vi "烧录座设定界面.vi"(8 "错误输入（无错误）":errorcluster, 10 "界面切换队列":refnum<queue>, 11 "VISA资源名称输入":refnum<visa-resource-name>) -> (0 "错误输出":errorcluster, 3 "VISA资源名称输出":refnum<visa-resource-name>)   [LabVIEW 2018]
panel:
  out "毫秒计时值":u32
  in  "枚举":T1(ring)
  in  "选项卡控件":enum32{"选项卡 1", "选项卡 2"}(tab)
  out "烧录座显示界面":bool
  out "读DDT32670+写R57F":dbl
  out "读DDT32668+写R57E":dbl
  out "读DDT32666+写R57D":dbl
  out "读DDT32664+写R57C":dbl
  out "读DDT32662+写R57B":dbl
  out "读DDT32660+写R57A":dbl
  out "读DDT32658+写R579":dbl
  out "读DDT32656+写R578":dbl
  out "读DDT32654+写R577":dbl
  out "读DDT32652+写R576":dbl
  out "读DDT32650+写R575":dbl
  out "读DDT32648+写R574":dbl
  out "读DDT32646+写R573":dbl
  out "读DDT32644+写R572":dbl
  out "读DDT32642+写R571":dbl
  out "读DDT32640+写R570":dbl
  out "写DDT32569":dbl
  out "写DDT32594":dbl
  out "DDT90356":dbl
  out "DDT90348":dbl
  out "自动界面":bool
  out "手动界面":bool
  out "参数界面":bool
  out "IO界面":bool
  out "产品界面":bool
  out "字符串":string
  out "DDT90352":dbl
  out "DDT90360":dbl
  out "通讯周期":dbl
  out "DT1184":T2(ring)
  # "X"
  # "Z1"
  # "Z2"
  # "Y"
  # "烧录座使用寿命"
  # "次"
  # "次"
  # "烧录座连续NG次数"
  # "烧录座当前烧录次数"
  # "1"
  # "2"
  # "3"
  # "4"
  # "5"
  # "6"
  # "7"
  # "8"
  # "9"
  # "10"
  # "12"
  # "14"
  # "15"
  # "16"
  # "11"
  # "13"
  # "鼠标点击数值框清零"
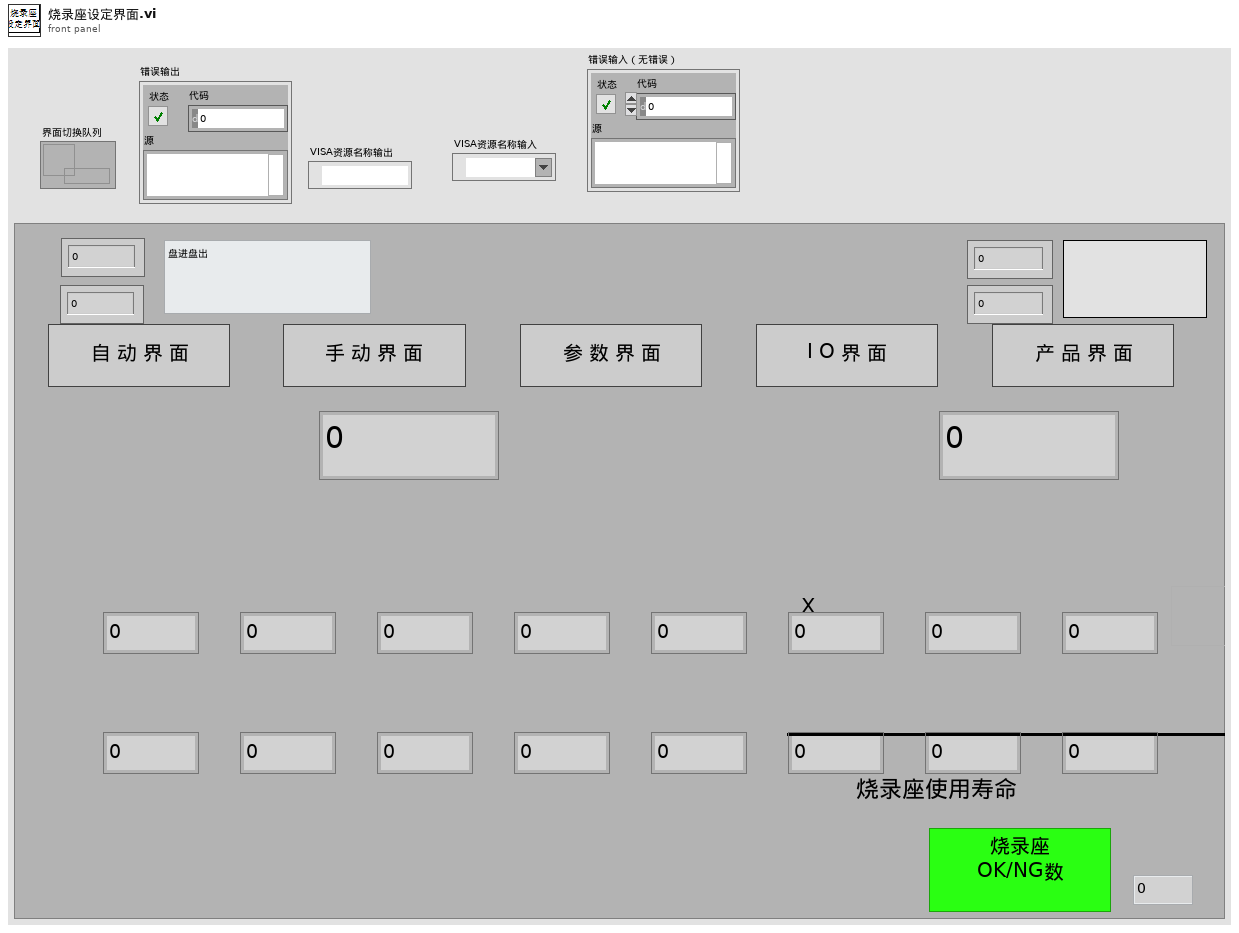
[diagram p1: front panel]
types:
  T1 = enum16{"读初始化", "读DDT32640+5", "读DDT32650+5", "读DDT32660+5", "读DDT32670", "读DDT32594", "读DDT32569", "读DDT90356", "读DT1184", "读DDT90348", ""}
  T2 = enum16{"盘进盘出", "卷进卷出", "盘进卷出", "管进盘出", "管进卷出", "卷进盘出", ""}
  T3 = enum8{"Enabled", "Disabled", "Disabled and Grayed Out"}
  T4 = typedef "数据簇.ctl" = cluster{"字符串":string, "数值":i32, "布尔":bool}
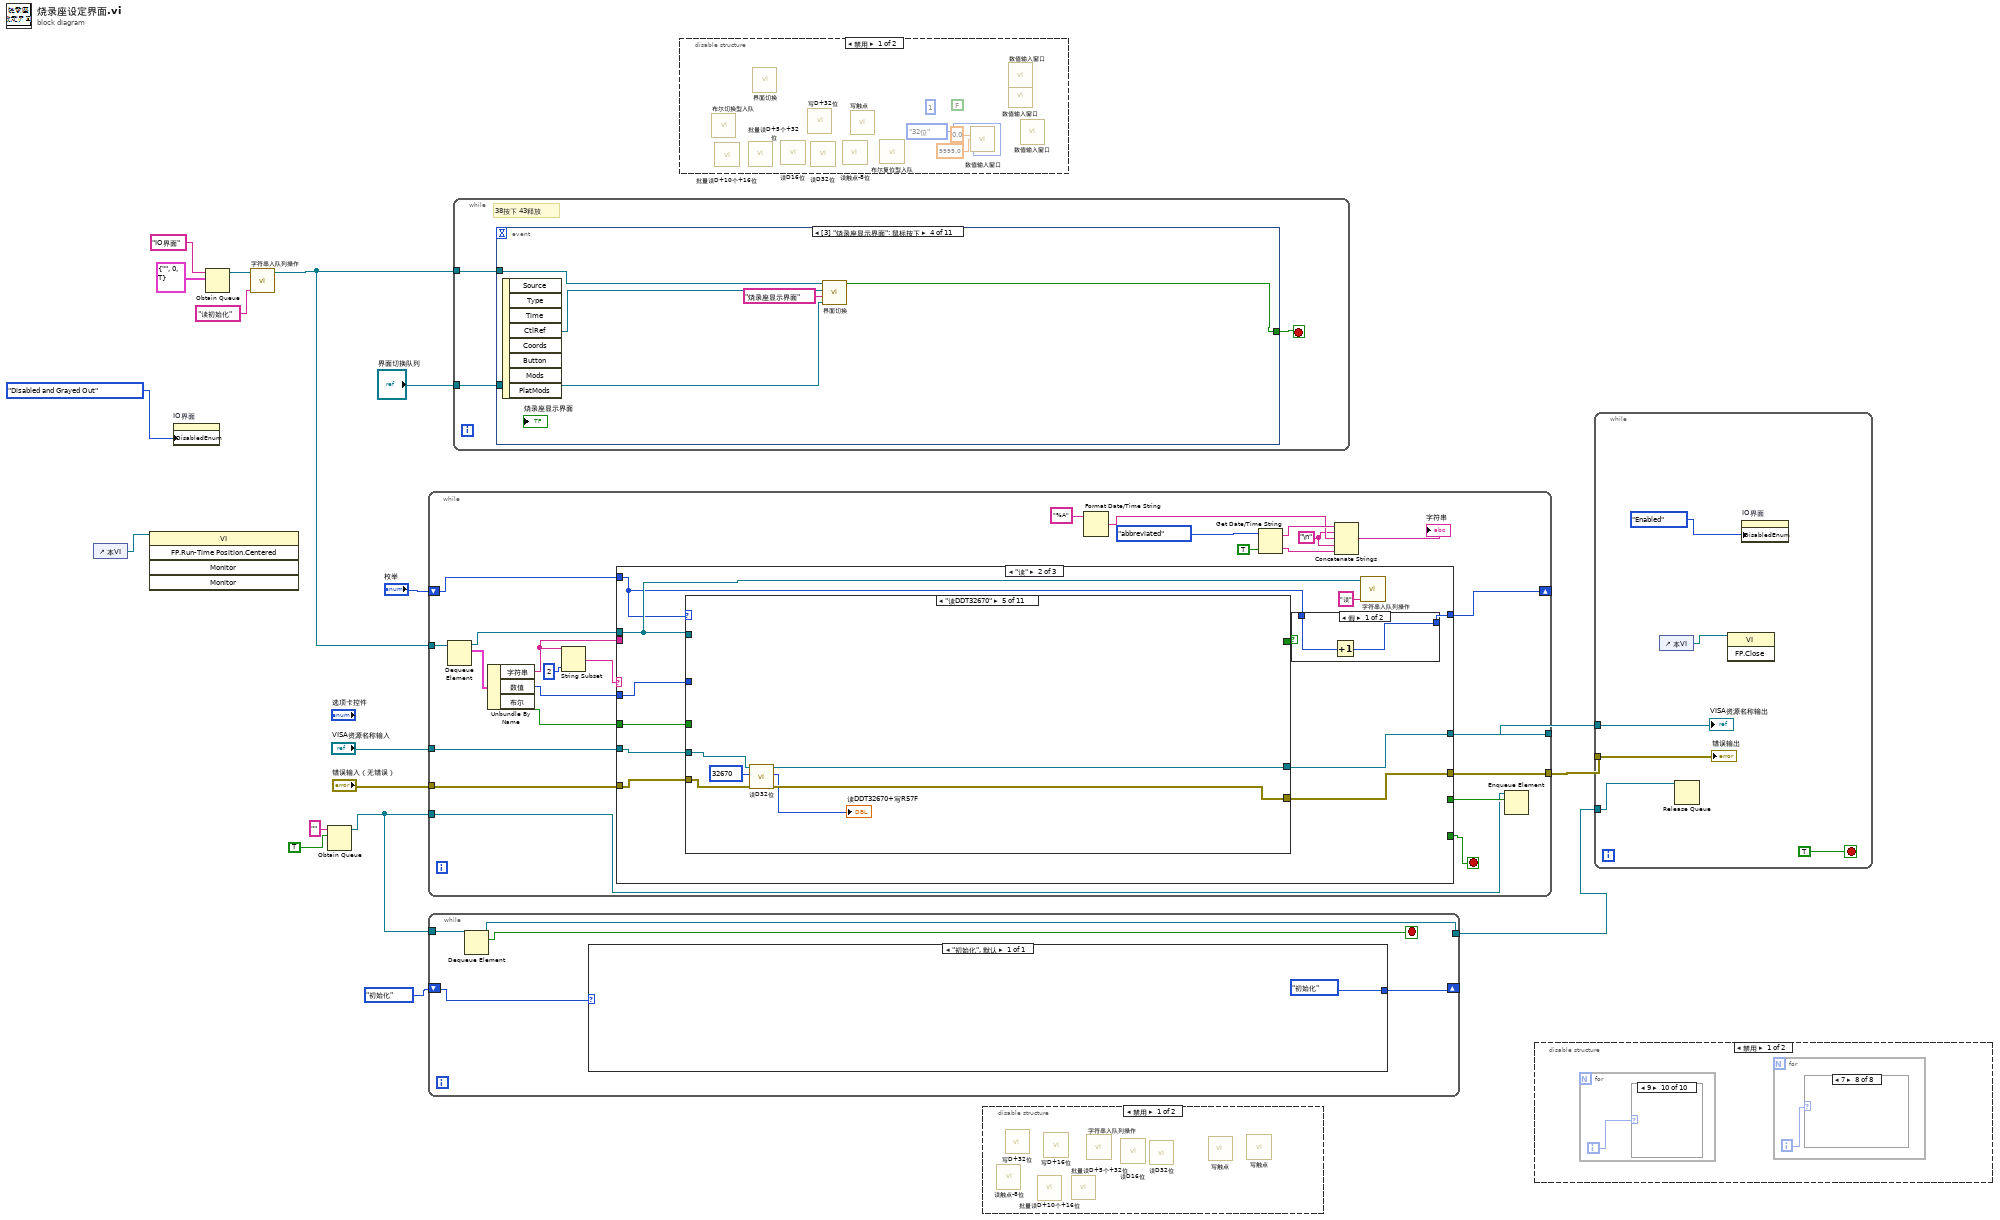
[diagram p0: block diagram]
diagram:
  n1 = control-ref of="本VI"() -> (w1:refnum<vi>)
  n2 = invoke class="VI" method="FP.Run-Time Position.Centered"(reference=w1) -> ()  [unwired: 4 in, 5 out]
  n3 = property on="IO界面" class="Bool"("DisabledEnum"=T3."Disabled and Grayed Out" ("禁用")) -> ()  [unwired: 2 in, 2 out]
  n4 = Obtain Queue(name (unnamed)="IO界面" ("名称（未命名）"), element data type=T4 {"字符串"="", "数值"=0, "布尔"=TRUE}) -> (queue out=w11:refnum<queue>)  [unwired: 3 in, 2 out]
  n5 = call "字符串入队列操作.vi"("字符消息入队列"="读初始化", "界面切换队列"=w11) -> ("队列输出"=w3:refnum<queue>)  [unwired: 9 in]
  n6 = Obtain Queue(name (unnamed)="" ("名称（未命名）"), element data type=TRUE) -> (queue out=w6:refnum<queue>)  [unwired: 3 in, 2 out]
  n7 = while {
    tunnel: w3 -> [w39]
    tunnel: "VISA资源名称输入" -> [w32]
    tunnel: "错误输入（无错误）" -> [w31]
    tunnel: [w30] -> w13
    tunnel: [w29] -> w12
    shift-right: [w26] -> _
    shift-left: "枚举" -> [w27]
    tunnel: w6 -> [w19]
    stop <- w21 stop-if-true
    w23 = "\n"
    n8 = Dequeue Element(queue=w39) -> (queue out=w36:refnum<queue>, element=w38:T4)  [unwired: 2 in, 2 out]
    n9 = Unbundle By Name(w38) -> ("字符串"=w33:string, "数值"=w35:i32, "布尔"=w34:bool)
    n10 = String Subset(string=w33, length (rest)=2 ("长度（剩余）")) -> (substring=w37:string)  [unwired: 1 in]
    n11 = case shown="\"读\"" w37 {
      selector: w37 -> [w46 _ _]
      tunnel: w36 -> [_ w54 w180]
      tunnel: w35 -> [_ w61 w179]
      tunnel: w34 -> [_ w60 w178]
      tunnel: w33 -> [_ _ w172]
      tunnel: w32 -> [w45 w59 w177]
      tunnel: w31 -> [w44 w58 w176]
      tunnel: [w45 w57 w174] -> w30
      tunnel: [w44 w56 w173] -> w29
      tunnel: [_ _ w175] -> w21
      tunnel: w27 -> [_ w52 _]
      tunnel: [_ w51 _] -> w26
      tunnel: [_ _ w170] -> w20
      frame "", Default {
        n12 = Concatenate Strings("无对应消息分支**" ("消息"), w46, "**" ("字符串"), "读写状态机" ("字符串")) -> (w48:string)
        n13 = One Button Dialog(message=w48) -> ()  [unwired: 1 in, 1 out]
      }
      frame "读" {
        n14 = case shown="\"读DDT32670\"" w52 {
          tunnel: w54 -> [_ _ _ _ _ _ _ _ _ _ _]
          tunnel: w61 -> [_ _ _ _ _ _ _ _ _ _ _]
          tunnel: w59 -> [w66 w72 w85 w98 w111 w117 w123 w135 w144 w157 w169]
          tunnel: w58 -> [w65 w71 w84 w97 w110 w116 w122 w134 w143 w156 w168]
          tunnel: [w66 w70 w83 w95 w109 w115 w120 w133 w142 w155 w169] -> w57
          tunnel: [w65 w69 w82 w94 w108 w114 w119 w132 w141 w154 w168] -> w56
          tunnel: w60 -> [_ _ _ _ _ _ _ _ _ _ _]
          tunnel: [_ _ _ _ _ _ _ _ _ _ TRUE] -> w53
          frame "读初始化" {
            n15 = Tick Count (ms)() -> (millisecond timer value=→"毫秒计时值":u32)
          }
          frame "读DDT32640+5" {
            n16 = call "批量读D+5个+32位.vi"("error out"=w71, "读取D地址"=32640, "VISA resource name out"=w72) -> ("error IO"=w69:errorcluster, "数组"=w67:i32[], "VISA resource name out 2"=w70:refnum<visa-resource-name>)  [unwired: 5 in, 1 out]
            n17 = for {
              tunnel: w67 -> [w73] mode=indexing
              i -> [w74]
              n18 = case shown="4" w74 {
                tunnel: w73 -> [w75 w76 w77 w78 w79]
                frame 0, Default {
                  "读DDT32640+写R570" <- w75
                }
                frame 1 {
                  "读DDT32642+写R571" <- w76
                }
                frame 2 {
                  "读DDT32644+写R572" <- w77
                }
                frame 3 {
                  "读DDT32646+写R573" <- w78
                }
                frame 4 {
                  "读DDT32648+写R574" <- w79
                }
              }
            }
          }
          frame "读DDT32650+5" {
            n19 = call "批量读D+5个+32位.vi"("error out"=w84, "读取D地址"=32650, "VISA resource name out"=w85) -> ("error IO"=w82:errorcluster, "数组"=w80:i32[], "VISA resource name out 2"=w83:refnum<visa-resource-name>)  [unwired: 5 in, 1 out]
            n20 = for {
              tunnel: w80 -> [w86] mode=indexing
              i -> [w87]
              n21 = case shown="3" w87 {
                tunnel: w86 -> [w88 w89 w90 w91 w92]
                frame 0, Default {
                  "读DDT32650+写R575" <- w88
                }
                frame 1 {
                  "读DDT32652+写R576" <- w89
                }
                frame 2 {
                  "读DDT32654+写R577" <- w90
                }
                frame 3 {
                  "读DDT32656+写R578" <- w91
                }
                frame 4 {
                  "读DDT32658+写R579" <- w92
                }
              }
            }
          }
          frame "读DDT32660+5" {
            n22 = call "批量读D+5个+32位.vi"("error out"=w97, "读取D地址"=32660, "VISA resource name out"=w98) -> ("error IO"=w94:errorcluster, "数组"=w93:i32[], "VISA resource name out 2"=w95:refnum<visa-resource-name>)  [unwired: 5 in, 1 out]
            n23 = for {
              tunnel: w93 -> [w99] mode=indexing
              i -> [w100]
              n24 = case shown="0, 默认" w100 {
                tunnel: w99 -> [w101 w102 w103 w104 w105]
                frame 0, Default {
                  "读DDT32660+写R57A" <- w101
                }
                frame 1 {
                  "读DDT32662+写R57B" <- w102
                }
                frame 2 {
                  "读DDT32664+写R57C" <- w103
                }
                frame 3 {
                  "读DDT32666+写R57D" <- w104
                }
                frame 4 {
                  "读DDT32668+写R57E" <- w105
                }
              }
            }
          }
          frame "读DDT32670" {
            n25 = call "读D32位.vi"("error out"=w110, "读取D地址"=32670, "VISA resource name out"=w111) -> ("error IO"=w108:errorcluster, "数值"=→"读DDT32670+写R57F":i32, "VISA resource name out 2"=w109:refnum<visa-resource-name>)  [unwired: 6 in]
          }
          frame "读DDT32594" {
            n26 = call "读D32位.vi"("error out"=w116, "读取D地址"=32594, "VISA resource name out"=w117) -> ("error IO"=w114:errorcluster, "数值"=→"写DDT32594":i32, "VISA resource name out 2"=w115:refnum<visa-resource-name>)  [unwired: 6 in]
          }
          frame "读DDT32569" {
            n27 = call "读D32位.vi"("error out"=w122, "读取D地址"=32569, "VISA resource name out"=w123) -> ("error IO"=w119:errorcluster, "数值"=→"写DDT32569":i32, "VISA resource name out 2"=w120:refnum<visa-resource-name>)  [unwired: 6 in]
          }
          frame "读DDT90356" {
            n28 = call "批量读D+5个+32位.vi"("error out"=w134, "读取D地址"=90356, "VISA resource name out"=w135) -> ("error IO"=w132:errorcluster, "数组"=w138:i32[], "VISA resource name out 2"=w133:refnum<visa-resource-name>)  [unwired: 5 in, 1 out]
            n29 = Index Array(array=w138, index #1=0 ("索引"), index #2=2 ("索引")) -> (element #1=w131:i32, element #2=w130:i32)
            n30 = To Double Precision Float(number=w131) -> (double precision float=w129:dbl)
            n31 = To Double Precision Float(number=w130) -> (double precision float=w126:dbl)
            n32 = Divide(x=w129, y=100.0) -> (x/y=→"DDT90356":dbl)
            n33 = Divide(x=w126, y=100.0) -> (x/y=→"DDT90360":dbl)
          }
          frame "读DT1184" {
            n34 = call "读D16位.vi"("error out"=w143, "读取D地址"=1184, "VISA resource name out"=w144) -> ("error IO"=w141:errorcluster, "数值"=→"DT1184":u32, "VISA resource name out 2"=w142:refnum<visa-resource-name>)  [unwired: 5 in, 1 out]
          }
          frame "读DDT90348" {
            n35 = call "批量读D+5个+32位.vi"("error out"=w156, "读取D地址"=90348, "VISA resource name out"=w157) -> ("error IO"=w154:errorcluster, "数组"=w161:i32[], "VISA resource name out 2"=w155:refnum<visa-resource-name>)  [unwired: 5 in, 1 out]
            n36 = Index Array(array=w161, index #1=0 ("索引"), index #2=2 ("索引")) -> (element #1=w153:i32, element #2=w152:i32)
            n37 = To Double Precision Float(number=w152) -> (double precision float=w147:dbl)
            n38 = To Double Precision Float(number=w153) -> (double precision float=w151:dbl)
            n39 = Divide(x=w147, y=100.0) -> (x/y=→"DDT90352":dbl)
            n40 = Divide(x=w151, y=100.0) -> (x/y=→"DDT90348":dbl)
          }
          frame "" {
            n41 = local read "毫秒计时值"() -> (w165:u32)
            n42 = Tick Count (ms)() -> (millisecond timer value=w166:u32)
            n43 = Subtract(x=w166, y=w165) -> (x-y=w164:u32)
            n44 = Divide(x=w164, y=u32 1000) -> (x/y=→"通讯周期":dbl)
          }
        }
        n45 = case shown="假" w53 {
          tunnel: w52 -> [w63 _]
          tunnel: [w62 _] -> w51
          frame False {
            n46 = Increment(x=w63) -> (x+1=w62:T1)
          }
          frame True {
          }
        }
        n47 = call "字符串入队列操作.vi"("字符消息入队列"="读", "界面切换队列"=w54) -> ()  [unwired: 9 in, 1 out]
      }
      frame "写" {
        n48 = call "状态匹配.vi"("输入状态"=w172) -> ("输出状态"=w171:string)  [unwired: 10 in]
        n49 = case shown="\"写退出\"" w171 {
          selector: w171 -> [w183 _ _ _ _]
          tunnel: w180 -> [_ _ _ _ w223]
          tunnel: w179 -> [_ w189 w206 _ _]
          tunnel: w178 -> [_ _ _ w217 _]
          tunnel: w177 -> [w182 w199 w210 w222 w228]
          tunnel: w176 -> [w181 w198 w209 w221 w227]
          tunnel: [_ _ _ _ w226] -> w175
          tunnel: [w182 w197 w208 w220 w228] -> w174
          tunnel: [w181 w196 w207 w219 w227] -> w173
          tunnel: w172 -> [_ w188 w200 w211 _]
          tunnel: [_ _ _ _ w226] -> w170
          frame "", Default {
            n50 = Concatenate Strings("无对应消息分支**" ("消息"), w183, "**" ("字符串"), "写状态机" ("字符串")) -> (w187:string)
            n51 = One Button Dialog(message=w187) -> ()  [unwired: 1 in, 1 out]
          }
          frame "写DT" {
            n52 = String Length(string=w188) -> (length=w194:i32)
            n53 = Subtract(x=w194, y=4) -> (x-y=w192:i32)
            n54 = String Subset(string=w188, offset (0)=4 ("偏移量(0)"), length (rest)=w192) -> (substring=w191:string)
            n55 = Decimal String To Number(string=w191) -> (number=w190:i32)  [unwired: 2 in, 1 out]
            n56 = call "写D+16位.vi"("error out"=w198, "输入数值"=w189, "输入地址D"=w190, "VISA resource name out"=w199) -> ("error out 2"=w196:errorcluster, "VISA resource name out 2"=w197:refnum<visa-resource-name>)  [unwired: 3 in, 3 out]
          }
          frame "写DDT" {
            n57 = String Length(string=w200) -> (length=w204:i32)
            n58 = Subtract(x=w204, y=5) -> ()  [unwired: 1 out]
            n59 = String Subset(string=w200, offset (0)=5 ("偏移量(0)")) -> (substring=w201:string)  [unwired: 1 in]
            n60 = Decimal String To Number(string=w201) -> (number=w202:i32)  [unwired: 2 in, 1 out]
            n61 = call "写D+32位.vi"("error out"=w209, "输入数值"=w206, "输入地址D"=w202, "VISA resource name out"=w210) -> ("error out 2"=w207:errorcluster, "VISA resource name out 2"=w208:refnum<visa-resource-name>)  [unwired: 4 in, 2 out]
          }
          frame "写R" {
            n62 = String Length(string=w211) -> (length=w215:i32)
            n63 = Subtract(x=w215, y=3) -> (x-y=w213:i32)
            n64 = String Subset(string=w211, offset (0)=3 ("偏移量(0)"), length (rest)=w213) -> (substring=w212:string)
            n65 = call "写触点.vi"("布尔"=w217, "error out"=w221, "触点类型"="R", "写入起始地址"=w212, "VISA resource name out"=w222) -> ("error IO"=w219:errorcluster, "VISA resource name out 2"=w220:refnum<visa-resource-name>)  [unwired: 4 in, 1 out]
          }
          frame "写退出" {
            w226 = TRUE
            n66 = Flush Queue(queue=w223) -> (queue out=w224:refnum<queue>, error out=w225:errorcluster)  [unwired: 1 in, 1 out]
            n67 = Release Queue(queue=w224, error in (no error)=w225) -> ()  [unwired: 1 in, 3 out]
          }
        }
      }
    }
    n68 = Format Date/Time String(time format string (%c)="%A" ("时间格式字符串(%c)")) -> (date/time string=w24:string)  [unwired: 2 in]
    n69 = Get Date/Time String(date format (0)=enum16{"short", "long", "abbreviated"}."abbreviated" ("日期格式(0)"), want seconds? (F)=TRUE ("需要秒？(F)")) -> (date string=w41:string, time string=w22:string)  [unwired: 1 in]
    n70 = Concatenate Strings(w41, w23, w24, w23, w22) -> (→"字符串":string)
    n71 = Enqueue Element(queue=w19, element=w20) -> ()  [unwired: 2 in, 3 out]
  }
  n72 = while {
    shift-right: [w232] -> _
    shift-left: enum16{"初始化"}."初始化" -> [w233]
    tunnel: w6 -> [w231]
    tunnel: [w229] -> w5
    stop <- w230 stop-if-true
    n73 = Dequeue Element(queue=w231) -> (queue out=w229:refnum<queue>, element=w230:bool)  [unwired: 2 in, 2 out]
    n74 = case shown="\"初始化\", 默认" w233 {
      tunnel: [enum16{"初始化"}."初始化"] -> w232
      frame "初始化", Default {
      }
    }
  }
  n75 = while {
    tunnel: w3 -> [w236]
    tunnel: "界面切换队列" -> [w235]
    stop <- w237 stop-if-true
    # "38按下 43释放"
    n76 = event shown="[3] \"烧录座显示界面\": 鼠标按下" {
      selector: _ -> [_ _ _ _ _ _ _ _ _ _ _]
      dyn-events: _ -> [_ _ _ _ _ _ _ _ _ _ _]
      timeout: _ -> [_ _ _ _ _ _ _ _ _ _ _]
      tunnel: [w241 w243 w248 w253 _ _ _ w296 w301 _ w308] -> w237
      tunnel: w236 -> [w242 w247 w252 w257 w265 w273 w277 w300 w305 _ w307]
      tunnel: w235 -> [w240 w246 w251 w255 _ _ _ w299 w304 _ w306]
      event "IO界面": Mouse Down {
        n77 = event-data() -> ("CtlRef"=w239:refnum<vi>)  [unwired: 1 in, 7 out]
        n78 = call "界面切换.vi"("界面切换队列输入"=w240, "切换界面名称输入"="IO界面", "Bool引用句柄"=w239, "状态转移输入"=w242) -> ("布尔"=w241:bool)  [unwired: 7 in]
      }
      event "参数界面": Mouse Down {
        n79 = event-data() -> ("CtlRef"=w245:refnum<vi>)  [unwired: 1 in, 7 out]
        n80 = call "界面切换.vi"("界面切换队列输入"=w246, "切换界面名称输入"="参数界面", "Bool引用句柄"=w245, "状态转移输入"=w247) -> ("布尔"=w243:bool)  [unwired: 7 in]
      }
      event "产品界面": Mouse Down {
        n81 = event-data() -> ("CtlRef"=w250:refnum<vi>)  [unwired: 1 in, 7 out]
        n82 = call "界面切换.vi"("界面切换队列输入"=w251, "切换界面名称输入"="产品界面", "Bool引用句柄"=w250, "状态转移输入"=w252) -> ("布尔"=w248:bool)  [unwired: 7 in]
      }
      event "烧录座显示界面": Mouse Down {
        n83 = event-data() -> ("CtlRef"=w256:refnum<vi>)  [unwired: 1 in, 7 out]
        n84 = call "界面切换.vi"("界面切换队列输入"=w255, "切换界面名称输入"="烧录座显示界面", "Bool引用句柄"=w256, "状态转移输入"=w257) -> ("布尔"=w253:bool)  [unwired: 7 in]
      }
      event "写DDT32594": Mouse Down {
        n85 = event-data() -> ("CtlRef"=w262:refnum<vi>)  [unwired: 1 in, 7 out]
        n86 = call "数值输入窗口.vi"("消息入队"=w265, "字符串"="烧录座使用寿命次数", "字符消息入队列"="写DDT32594", "输入下限"=0.0, "输入上限"=999999999.0, "转换比例"=u32 1, "数据类型"=enum16{"32位", "16位"}."32位", "控件引用"=w262) -> ()  [unwired: 5 in, 3 out]
      }
      event "写DDT32569": Mouse Down {
        n87 = event-data() -> ("CtlRef"=w270:refnum<vi>)  [unwired: 1 in, 7 out]
        n88 = call "数值输入窗口.vi"("消息入队"=w273, "字符串"="烧录座连续NG次数", "字符消息入队列"="写DDT32569", "输入下限"=0.0, "输入上限"=999999999.0, "转换比例"=u32 1, "数据类型"=enum16{"32位", "16位"}."32位", "控件引用"=w270) -> ()  [unwired: 5 in, 3 out]
      }
      event "读DDT32640+写R570", "读DDT32642+写R571", "读DDT32644+写R572", "读DDT32646+写R573", "读DDT32648+写R574", "读DDT32650+写R575", "读DDT32652+写R576", "读DDT32654+写R577", "读DDT32656+写R578", "读DDT32658+写R579", "读DDT32660+写R57A", "读DDT32662+写R57B", "读DDT32664+写R57C", "读DDT32666+写R57D", "读DDT32668+写R57E", "读DDT32670+写R57F": Mouse Down {
        n89 = event-data() -> ("CtlRef"=w279:refnum<vi>)  [unwired: 1 in, 7 out]
        n90 = property class="DigNum (严格)"(reference=w279) -> (reference out=w278:refnum<vi>, "Label.Text"=w276:string)  [unwired: 1 in, 1 out]
        n91 = Two Button Dialog(message="确定清零烧录次数?" ("消息")) -> (T button?=w280:bool)  [unwired: 2 in]
        n92 = Match Pattern(string=w276, regular expression="+" ("正则表达式")) -> (after substring=w274:string)  [unwired: 1 in, 3 out]
        n93 = case shown="真" w280 {
          tunnel: w278 -> [_ w290]
          tunnel: w277 -> [_ w292]
          tunnel: w274 -> [_ w291]
          frame False {
          }
          frame True {
            n94 = call "布尔复位型入队.vi"("队列输入"=w292, "数值"=38, "控件引用"=w290, "字符消息入队列"=w291) -> ("队列输出"=w288:refnum<queue>, "控件引用 2"=w287:refnum<vi>, "字符消息出队列"=w286:string)  [unwired: 2 in]
            n95 = flat-sequence {
              tunnel: w288 -> [w295]
              tunnel: w287 -> [w294]
              tunnel: w286 -> [w293]
              tunnel: [w295] -> w285
              tunnel: [w294] -> w284
              tunnel: [w293] -> w283
              frame #0 {
              }
            }
            n96 = call "布尔复位型入队.vi"("队列输入"=w285, "数值"=43, "控件引用"=w284, "字符消息入队列"=w283) -> ()  [unwired: 2 in, 3 out]
          }
        }
      }
      event "手动界面": Mouse Down {
        n97 = event-data() -> ("CtlRef"=w298:refnum<vi>)  [unwired: 1 in, 7 out]
        n98 = call "界面切换.vi"("界面切换队列输入"=w299, "切换界面名称输入"="手动界面", "Bool引用句柄"=w298, "状态转移输入"=w300) -> ("布尔"=w296:bool)  [unwired: 7 in]
      }
      event "自动界面": Mouse Down {
        n99 = event-data() -> ("CtlRef"=w303:refnum<vi>)  [unwired: 1 in, 7 out]
        n100 = call "界面切换.vi"("界面切换队列输入"=w304, "切换界面名称输入"="自动界面", "Bool引用句柄"=w303, "状态转移输入"=w305) -> ("布尔"=w301:bool)  [unwired: 7 in]
      }
      event Timeout {
        n101 = event-data() -> ()  [unwired: 1 in, 3 out]
      }
      event Panel Close? {
        n102 = event-data() -> ()  [unwired: 1 in, 4 out]
        n103 = Two Button Dialog(message="确定退出程序？" ("消息")) -> (T button?=w309:bool)  [unwired: 2 in]
        n104 = case shown="真" w309 {
          tunnel: [_ TRUE] -> w308
          tunnel: w307 -> [_ w314]
          tunnel: w306 -> [_ w313]
          frame False {
          }
          frame True {
            n105 = call "字符串入队列操作.vi"("字符消息入队列"="退出", "界面切换队列"=w313) -> ()  [unwired: 9 in, 1 out]
            n106 = call "字符串入队列操作.vi"("字符消息入队列"="写退出", "界面切换队列"=w314) -> ()  [unwired: 9 in, 1 out]
          }
        }
        n107 = event-data("Discard?"=TRUE ("放弃？")) -> ()  [unwired: 1 in, 1 out]
      }
    }
  }
  n108 = disable-structure shown="禁用" {
    frame Disabled {
      (unwired) u32 1 ("转换比例")
      (unwired) FALSE ("忽略数值上下限")
      n109 = call "布尔切换型入队.vi"() -> ()  [unwired: 12 in]
      n110 = call "批量读D+10个+16位.vi"() -> ()  [unwired: 8 in, 4 out]
      n111 = call "批量读D+5个+32位.vi"() -> ()  [unwired: 8 in, 4 out]
      n112 = call "界面切换.vi"() -> ()  [unwired: 11 in, 1 out]
      n113 = call "读D16位.vi"() -> ()  [unwired: 8 in, 4 out]
      n114 = call "写D+32位.vi"() -> ()  [unwired: 8 in, 4 out]
      n115 = call "读D32位.vi"() -> ()  [unwired: 9 in, 3 out]
      n116 = call "读触点-8位.vi"() -> ()  [unwired: 8 in, 4 out]
      n117 = call "写触点.vi"() -> ()  [unwired: 9 in, 3 out]
      n118 = call "布尔复位型入队.vi"() -> ()  [unwired: 6 in, 3 out]
      n119 = call "数值输入窗口.vi"("输入下限"=0.0, "输入上限"=9999.0, "数据类型"=enum16{"32位", "16位"}."32位") -> ("转换比例"=w320:u32)  [unwired: 9 in, 3 out]
      n120 = call "数值输入窗口.vi"() -> ()  [unwired: 13 in, 3 out]
      n121 = call "数值输入窗口.vi"() -> ()  [unwired: 13 in, 3 out]
      n122 = call "数值输入窗口.vi"() -> ()  [unwired: 13 in, 3 out]
    }
    frame Enabled {
    }
  }
  n123 = disable-structure shown="禁用" {
    frame Disabled {
      n124 = call "读触点-8位.vi"() -> ()  [unwired: 8 in, 4 out]
      n125 = call "写D+32位.vi"() -> ()  [unwired: 8 in, 4 out]
      n126 = call "批量读D+10个+16位.vi"() -> ()  [unwired: 8 in, 4 out]
      n127 = call "写D+16位.vi"() -> ()  [unwired: 7 in, 5 out]
      n128 = call "批量读D+5个+32位.vi"() -> ()  [unwired: 8 in, 4 out]
      n129 = call "字符串入队列操作.vi"() -> ()  [unwired: 11 in, 1 out]
      n130 = call "读D16位.vi"() -> ()  [unwired: 8 in, 4 out]
      n131 = call "读D32位.vi"() -> ()  [unwired: 9 in, 3 out]
      n132 = call "写触点.vi"() -> ()  [unwired: 9 in, 3 out]
      n133 = call "写触点.vi"() -> ()  [unwired: 9 in, 3 out]
    }
    frame Enabled {
    }
  }
  n134 = disable-structure shown="禁用" {
    frame Disabled {
      n135 = for {
        i -> [w322]
        n136 = case shown="9" w322 {
          frame 0, Default {
          }
          frame 1 {
          }
          frame 2 {
          }
          frame 3 {
          }
          frame 4 {
          }
          frame 5 {
          }
          frame 6 {
          }
          frame 7 {
          }
          frame 8 {
          }
          frame 9 {
          }
        }
      }
      n137 = for {
        i -> [w321]
        n138 = case shown="7" w321 {
          frame 0, Default {
          }
          frame 1 {
          }
          frame 2 {
          }
          frame 3 {
          }
          frame 4 {
          }
          frame 5 {
          }
          frame 6 {
          }
          frame 7 {
          }
        }
      }
    }
    frame Enabled {
    }
  }
  n139 = while {
    tunnel: w13 -> [w326]
    tunnel: w12 -> [w325]
    tunnel: w5 -> [w324]
    stop <- TRUE stop-if-true
    n140 = control-ref of="本VI"() -> (w327:refnum<vi>)
    n141 = Release Queue(queue=w324) -> ()  [unwired: 2 in, 3 out]
    n142 = invoke class="VI" method="FP.Close"(reference=w327) -> ()  [unwired: 2 in, 3 out]
    n143 = property on="IO界面" class="Bool"("DisabledEnum"=T3."Enabled" ("禁用")) -> ()  [unwired: 2 in, 2 out]
    "VISA资源名称输出" <- w326
    "错误输出" <- w325
  }
